vi "KE_Reverse.vi"(7 "Boolean":bool=TRUE, 8 "error in (no error)":errorcluster, 11 "Instruments in":refnum<class "Instruments.lvclass">) -> (0 "error out":errorcluster, 2 "Current":dbl, 3 "Instruments out":refnum<class "Instruments.lvclass">)   [LabVIEW 2012, in "Instruments.lvclass"]
uses:
  Instruments.lvclass
  Instruments.lvclass/Instruments.ctl
  Instruments/Drivers/ke236/KE236.LLB/Keith 236 Operate/Standby.vi
panel:
  in  "integration time (medium:1)":u16(ring)=1 items=["fast perod", "medium period", "line cycle period @ 50Hz", "line cycle period @ 60Hz"]
  out "device dependent errors":string
  out "?":T1(array[cluster])
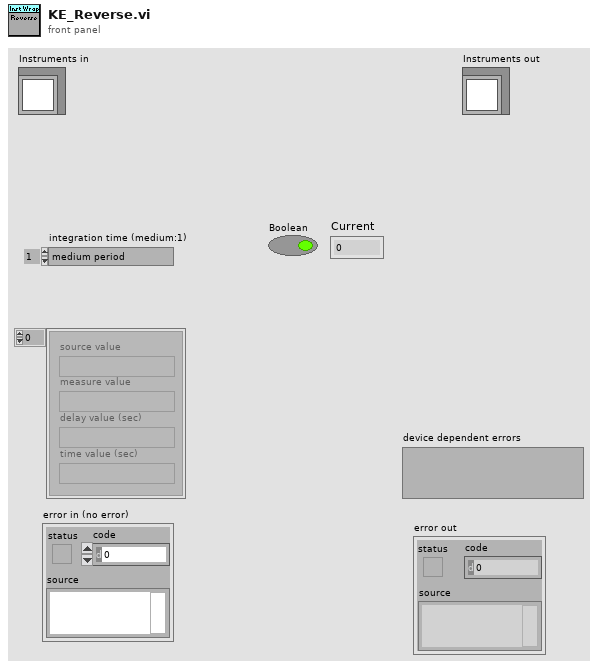
[diagram p1: front panel]
types:
  T1 = cluster{"source value":string, "measure value":string, "delay value (sec)":string, "time value (sec)":string}[]
  T2 = cluster{"Start Current,mA":dbl, "Stop Current,mA":dbl, "Voltage Compliance,V":dbl, "GPIB":string}
  T3 = cluster{"error":bool, "code":i32, "source":string}
  T4 = cluster{"source value":string, "measure value":string, "delay value (sec)":string, "time value (sec)":string}
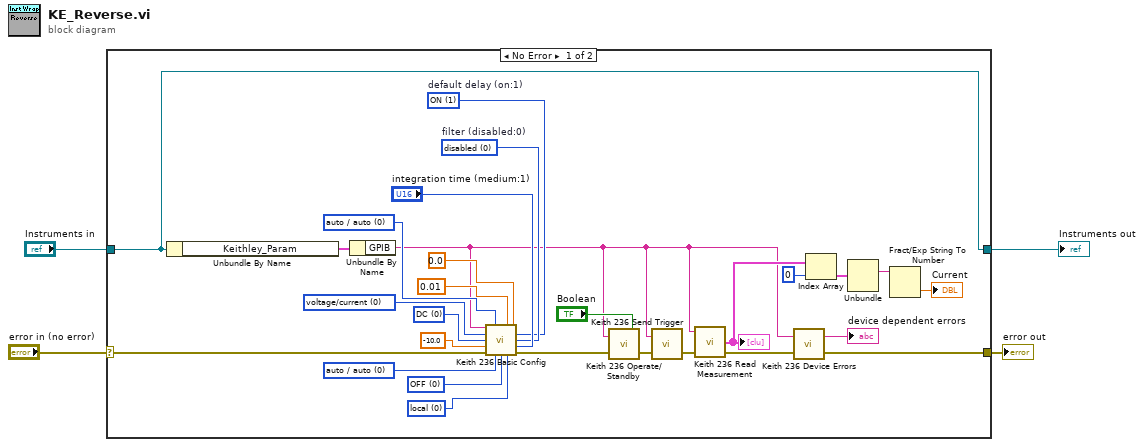
[diagram p0: block diagram]
diagram:
  n1 = case shown="No Error" "error in (no error)" {
    selector: "error in (no error)" -> [w8 w34]
    tunnel: [w9 w34] -> w3
    tunnel: [w6 w33] -> w1
    tunnel: "Instruments in" -> [w6 w33]
    frame No Error {
      w17 = u16 1 items=["OFF", "ON"]  # default delay (on:1)
      w18 = u16 0 items=["disabled", "2 readings", "4 readings", "8 readings", "16 readings", "32 readings"]  # filter (disabled:0)
      w21 = u16 0 items=["local", "remote"] ("sense (local:0)")
      w22 = u16 0 items=["OFF", "ON"] ("suppression (off:0)")
      w23 = u16 0 items=["auto / auto", "1 nA / 1.1 V", "10 nA / 11 V", "100 nA / 110 V", "0.001 mA / 110 V", "0.01 mA / 110 V", "0.1 mA / 110 V", "1 mA / 110 V", "10 mA / 110 V", "100 mA / 110 V"] ("compliance/\nmeasurement range (auto:0)")
      w24 = u16 0 items=["DC", "sweep"] ("function (DC:0)")
      w25 = u16 0 items=["voltage/current", "current/voltage"] ("source/measure (V/I:0)")
      w26 = u16 0 items=["auto / auto", "1 nA / 1.1 V", "10 nA / 11 V", "100 nA / 110 V", "0.001 mA / 110 V", "0.01 mA / 110 V", "0.1 mA / 110 V", "1 mA / 110 V", "10 mA / 110 V", "100 mA / 110 V"] ("source range\nI source / V source (auto:0)")
      n2 = Unbundle By Name(w6) -> ("Keithley_Param"=w32:T2)
      n3 = Unbundle By Name(w32) -> ("GPIB"=w5:string)
      n4 = call "Keith 236 Basic Config.vi"("GPIB address"=w5, "source range\nI source / V source (auto:0)"=w26, "current \ncompliance level"=0.01 ("current \ncompliance level"), "DC delay (sec)"=0.0, "source/measure (V/I:0)"=w25, "default delay (on:1)"=w17, "function (DC:0)"=w24, "filter (disabled:0)"=w18, "source level"=-10.0, "integration time (medium:1)"="integration time (medium:1)", "error in"=w8, "compliance/\nmeasurement range (auto:0)"=w23, "suppression (off:0)"=w22, "sense (local:0)"=w21) -> ("error out"=w16:T3)  [unwired: 1 in]
      n5 = call "Keith 236 Operate/Standby.vi"("source"="Boolean", "error in"=w16, "GPIB address"=w5) -> ("error out"=w28:T3)
      n6 = call "Keith 236 Send Trigger.vi"("GPIB address"=w5, "error in"=w28) -> ("error out"=w30:T3)
      n7 = call "Keith 236 Read Measurement.vi"("error in"=w30, "GPIB address"=w5) -> ("error out"=w31:T3, "display"=w15:T1)  [unwired: 2 out]
      "?" <- w15
      n8 = call "Keith 236 Device Errors.vi"("error in"=w31, "GPIB address"=w5) -> ("error out"=w9:T3, "device dependent errors"=→"device dependent errors":string)
      n9 = Index Array(array=w15, index=0) -> (element=w13:T4)
      n10 = Unbundle(w13) -> ("measure value"=w12:string)  [unwired: 3 out]
      n11 = Fract/Exp String To Number(string=w12) -> (number=→"Current":dbl)  [unwired: 3 in, 1 out]
    }
    frame Error {
    }
  }
  "error out" <- w3
  "Instruments out" <- w1
